vi "Larva Direction Select.vi"(7 "Danger":bool, 9 "Target Direction":T1, 11 "Position ID":T2) -> (3 "Move Array Out":T1[](array[typedef]))   [LabVIEW 2017, in "AntFarm_MB.lvclass"]
uses:
  AntFarm_MB.lvclass
  Type Defs/Direction Enum.ctl
  TypeDefs/ENUM_Position ID.ctl
  Type Defs/SB Type Defs.lvlib
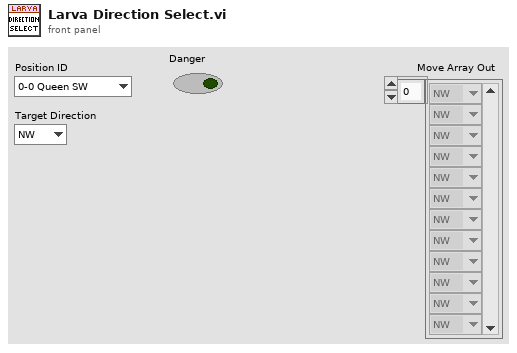
[diagram p1: front panel]
types:
  T1 = typedef "SB Type Defs.lvlib/Direction Enum.ctl" = enum16{"NW", "N", "NE", "E", "SE", "S", "SW", "W"}
  T2 = typedef "ENUM_Position ID.ctl" = enum16{"0-0 Queen SW", "0-1 Path E", "0-2 Queen NW", "0-3 Path W", "1-0 Path S", "1-1 Larva SW", "1-2 Path N", "1-3 Larva NW", "2-0 Queen SE", "2-1 Path W", "2-2 Queen NE", "2-3 Path E", "3-0 Path N", "3-1 Larva SE", "3-2 Path S", "3-3 Larva NE"}
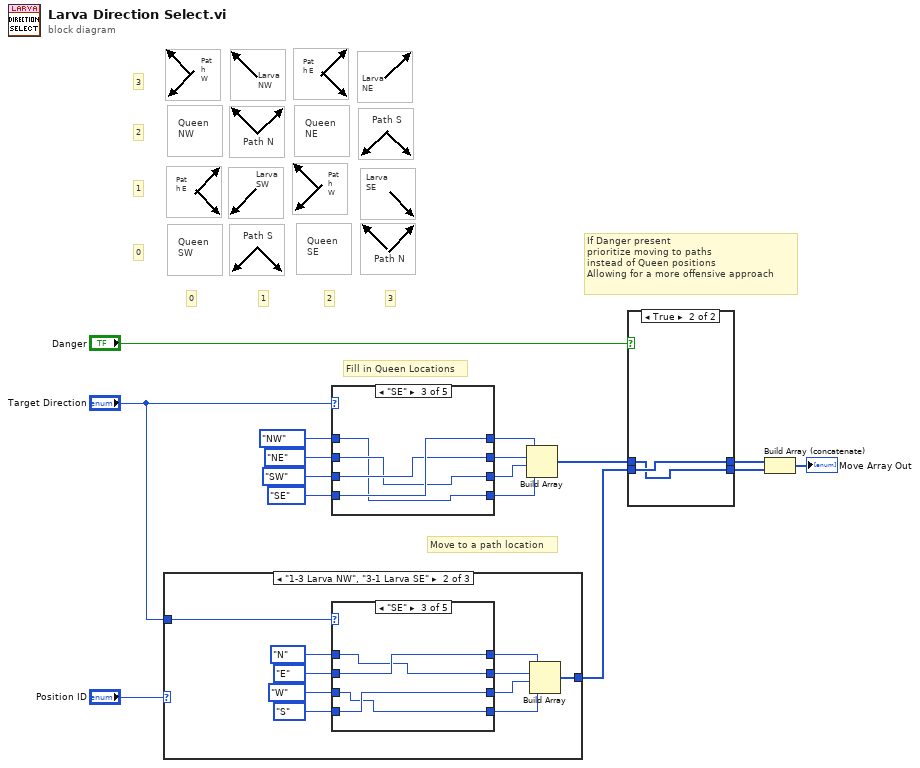
[diagram p0: block diagram]
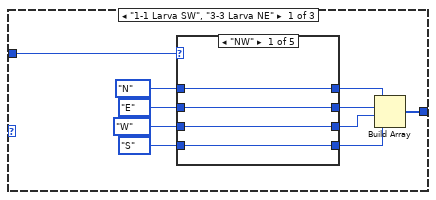
[diagram p7: hidden frame]
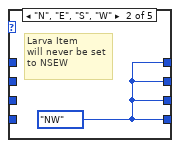
[diagram p8: hidden frame]
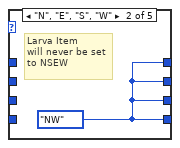
[diagram p13: hidden frame]
diagram:
  # "Path N"
  # "Path E"
  # "Path S"
  # "Path W"
  # "Path W"
  # "Path S"
  # "Path E"
  # "Path N"
  # "Larva\nNE"
  # "Larva\nSW"
  # "Larva\nNW"
  # "Queen\nNW"
  # "Queen\nNE"
  # "Queen\nSE"
  # "Larva\nSE"
  # "3"
  # "2"
  # "1"
  # "0"
  # "3"
  # "2"
  # "1"
  # "0"
  # "Queen\nSW"
  # "If Danger present\nprioritize moving to paths\ninstead of Queen positions\nAllowing for a more offensive approach"
  # "Move to a path location"
  # "Fill in Queen Locations"
  n1 = case shown="\"1-3 Larva NW\", \"3-1 Larva SE\"" "Position ID" {
    tunnel: "Target Direction" -> [w26 w53 _]
    tunnel: [w17 w44 _] -> w4
    frame "1-1 Larva SW", "3-3 Larva NE" {
      n2 = case shown="\"NW\"" w26 {
        tunnel: Direction_Enum."N" ("Primary Direction") -> [w30 _ w32 w36 w43]
        tunnel: Direction_Enum."E" ("Primary Direction") -> [w29 _ w33 w38 w41]
        tunnel: Direction_Enum."W" ("Primary Direction") -> [w28 _ w34 w37 w42]
        tunnel: Direction_Enum."S" ("Primary Direction") -> [w27 _ w35 w39 w40]
        tunnel: [w30 w31 w35 w39 w43] -> w21
        tunnel: [w29 w31 w34 w38 w42] -> w20
        tunnel: [w28 w31 w33 w37 w41] -> w19
        tunnel: [w27 w31 w32 w36 w40] -> w18
        frame "NW" {
        }
        frame "N", "E", "S", "W" {
          w31 = Direction_Enum."NW" ("Primary Direction")
          # "Larva Item\nwill never be set\nto NSEW"
        }
        frame "SE" {
        }
        frame "SW" {
        }
        frame "NE" {
        }
      }
      n3 = Build Array(w21, w20, w19, w18) -> (w17:T1[])
    }
    frame "1-3 Larva NW", "3-1 Larva SE" {
      n4 = case shown="\"SE\"" w53 {
        tunnel: Direction_Enum."N" ("Primary Direction") -> [w56 _ w61 w65 w68]
        tunnel: Direction_Enum."E" ("Primary Direction") -> [w54 _ w62 w63 w70]
        tunnel: Direction_Enum."W" ("Primary Direction") -> [w57 _ w59 w66 w67]
        tunnel: Direction_Enum."S" ("Primary Direction") -> [w55 _ w60 w64 w69]
        tunnel: [w57 w58 w62 w66 w70] -> w48
        tunnel: [w56 w58 w61 w65 w69] -> w47
        tunnel: [w55 w58 w60 w64 w68] -> w46
        tunnel: [w54 w58 w59 w63 w67] -> w45
        frame "NW" {
        }
        frame "N", "E", "S", "W" {
          w58 = Direction_Enum."NW" ("Primary Direction")
          # "Larva Item\nwill never be set\nto NSEW"
        }
        frame "SE" {
        }
        frame "SW" {
        }
        frame "NE" {
        }
      }
      n5 = Build Array(w48, w47, w46, w45) -> (w44:T1[])
    }
    frame Default {
      # "This vi is only\nfor Larva cases"
    }
  }
  n6 = case shown="\"SE\"" "Target Direction" {
    tunnel: Direction_Enum."NW" ("Primary Direction") -> [w74 w75 w76 w82 w85]
    tunnel: Direction_Enum."NE" ("Primary Direction") -> [w73 _ w77 w80 w87]
    tunnel: Direction_Enum."SW" ("Primary Direction") -> [w72 _ w78 w83 w84]
    tunnel: Direction_Enum."SE" ("Primary Direction") -> [w71 _ w79 w81 w86]
    tunnel: [w74 w75 w79 w83 w87] -> w7
    tunnel: [w73 w75 w78 w82 w86] -> w8
    tunnel: [w72 w75 w77 w81 w85] -> w9
    tunnel: [w71 w75 w76 w80 w84] -> w10
    frame "NW" {
    }
    frame "N", "E", "S", "W" {
      # "Larva Item\nwill never be set\nto NSEW"
    }
    frame "SE" {
    }
    frame "SW" {
    }
    frame "NE" {
    }
  }
  n7 = Build Array(w7, w8, w9, w10) -> (w5:T1[])
  n8 = case shown="True" "Danger" {
    tunnel: w5 -> [w89 w90]
    tunnel: w4 -> [w88 w91]
    tunnel: [w89 w91] -> w3
    tunnel: [w88 w90] -> w2
    frame False {
    }
    frame True {
    }
  }
  n9 = Build Array (concatenate)(w3, w2) -> (→"Move Array Out":T1[])
